vi "Handle getAll.vi"(8 "error in (no error)":errorcluster, 11 "instrument.Cryostation in":refnum<class "instrument.Cryostation.lvclass">) -> (0 "error out":errorcluster, 2 "getAll":variant, 3 "instrument.Cryostation out":refnum<class "instrument.Cryostation.lvclass">)   [LabVIEW 2019, in "instrument.Cryostation.lvclass"]
uses:
  instrument.Cryostation.lvclass
  instrument.Cryostation.lvclass/instrument.Cryostation.ctl
  Typedefs/Cryostation.getAll--cluster.ctl
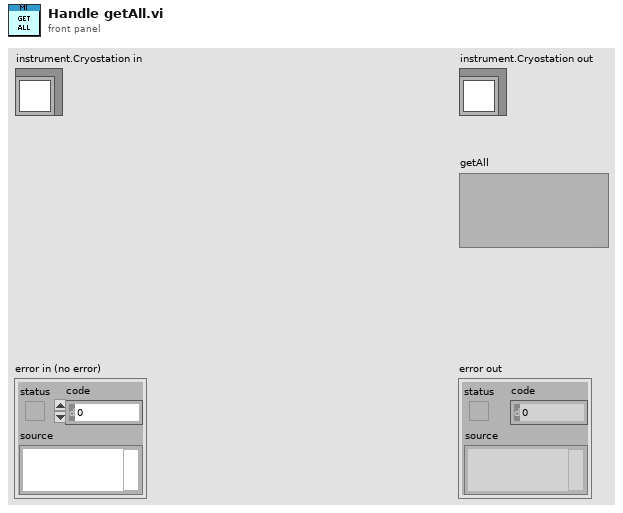
[diagram p1: front panel]
types:
  T1 = typedef "instrument.Cryostation.lvclass/Cryostation.getAll--cluster.ctl" = cluster{"Chamber Pressure (mTorr)":dbl, "Compressor Return Pressure (MPa)":dbl, "Compressor Supply Pressure (MPa)":dbl, "Compressor Speed (Hz)":dbl, "Cold Head Speed (Hz)":dbl, "Platform Heater Power (W)":dbl, "Platform Stability (K)":dbl, "Platform Temperature (K)":dbl, "Stage 1 Heater Power (W)":dbl, "Stage 1 Temperature (K)":dbl, "Stage 2 Heater Power (W)":dbl, "Stage 2 Temperature (K)":dbl, "Sample Stability (K)":dbl, "Sample Temperature (K)":dbl, "Temperature Set Point (K)":dbl, "User Stability (K)":dbl, "User Temperature (K)":dbl, "User Temperature Set Point (K)":dbl, "Alarm State":string, "Compressor Run State":string, "Case Valve State":string, "Idle State":string, "Nitrogen State":string, "Vent Valve State":string}
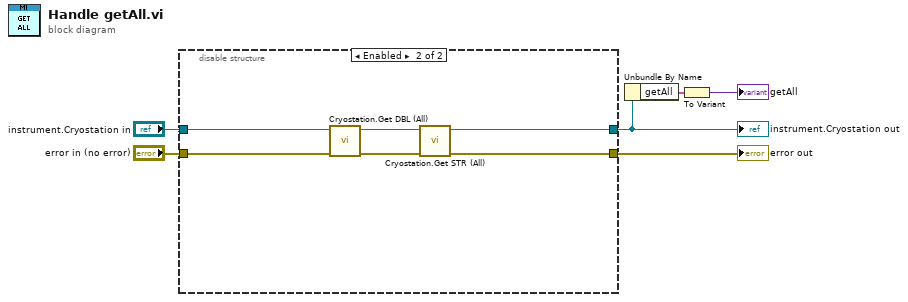
[diagram p0: block diagram]
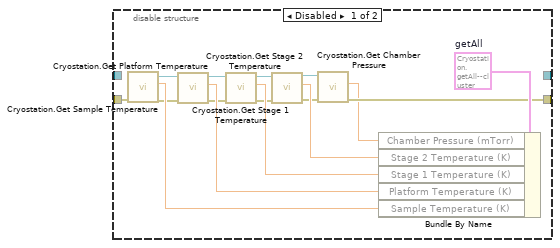
[diagram p2: hidden frame]
diagram:
  n1 = disable-structure shown="Enabled" {
    disable-tunnel: [w20 w24] -> w5
    disable-tunnel: "error in (no error)" -> [w21 w28]
    disable-tunnel: "instrument.Cryostation in" -> [_ w27]
    disable-tunnel: [_ w23] -> w1
    frame Disabled {
      w22 = T1 {"Chamber Pressure (mTorr)"=0.0, "Compressor Return Pressure (MPa)"=0.0, "Compressor Supply Pressure (MPa)"=0.0, "Compressor Speed (Hz)"=0.0, "Cold Head Speed (Hz)"=0.0, "Platform Heater Power (W)"=0.0, "Platform Stability (K)"=0.0, "Platform Temperature (K)"=0.0, "Stage 1 Heater Power (W)"=0.0, "Stage 1 Temperature (K)"=0.0, "Stage 2 Heater Power (W)"=0.0, "Stage 2 Temperature (K)"=0.0, "Sample Stability (K)"=0.0, "Sample Temperature (K)"=0.0, "Temperature Set Point (K)"=0.0, "User Stability (K)"=0.0, "User Temperature (K)"=0.0, "User Temperature Set Point (K)"=0.0, "Alarm State"="", "Compressor Run State"="", "Case Valve State"="", "Idle State"="", "Nitrogen State"="", "Vent Valve State"=""}  # getAll
      n2 = call "Cryostation.Get Sample Temperature.vi"("error in (no error)"=w21) -> ("error out"=w13:errorcluster, "Sample Temperature (K)"=w15:dbl, "TCP Network Connection out"=w14:refnum<k5>)  [unwired: 8 in]
      n3 = call "Cryostation.Get Platform Temperature.vi"("error in (no error)"=w13, "TCP Network Connection in"=w14) -> ("error out"=w11:errorcluster, "Platform Temperature (K)"=w16:dbl, "TCP Network Connection out"=w12:refnum<k5>)  [unwired: 7 in]
      n4 = call "Cryostation.Get Stage 1 Temperature.vi"("error in (no error)"=w11, "TCP Network Connection in"=w12) -> ("error out"=w9:errorcluster, "Stage 1 Temperature (K)"=w17:dbl, "TCP Network Connection out"=w10:refnum<k5>)  [unwired: 7 in]
      n5 = call "Cryostation.Get Stage 2 Temperature.vi"("error in (no error)"=w9, "TCP Network Connection in"=w10) -> ("error out"=w7:errorcluster, "Stage 2 Temperature (K)"=w18:dbl, "TCP Network Connection out"=w8:refnum<k5>)  [unwired: 7 in]
      n6 = call "Cryostation.Get Chamber Pressure.vi"("error in (no error)"=w7, "TCP Network Connection in"=w8) -> ("error out"=w20:errorcluster, "Chamber Pressure (mTorr)"=w19:dbl)  [unwired: 7 in, 1 out]
      n7 = Bundle By Name(cluster=w22, "Chamber Pressure (mTorr)"=w19, "Stage 2 Temperature (K)"=w18, "Stage 1 Temperature (K)"=w17, "Platform Temperature (K)"=w16, "Sample Temperature (K)"=w15) -> ()  [unwired: 1 out]
    }
    frame Enabled {
      n8 = call "Cryostation.Get DBL (All).vi"("error in (no error)"=w28, "instrument.Cryostation in"=w27) -> ("error out"=w25:errorcluster, "instrument.Cryostation out"=w26:refnum<class "instrument.Cryostation.lvclass">)  [unwired: 8 in]
      n9 = call "Cryostation.Get STR (All).vi"("error in (no error)"=w25, "instrument.Cryostation in"=w26) -> ("error out"=w24:errorcluster, "instrument.Cryostation out"=w23:refnum<class "instrument.Cryostation.lvclass">)  [unwired: 8 in]
    }
  }
  "error out" <- w5
  "instrument.Cryostation out" <- w1
  n10 = Unbundle By Name(w1) -> ("getAll"=w2:T1)
  n11 = To Variant(anything=w2) -> (Variant=→"getAll":variant)
